vi "set point count.vi"(8 "reset":bool, 9 "dt(s)":dbl, 10 "speed":dbl) -> (1 "setpoint":dbl)   [LabVIEW 2019, in "my FPGA lib.lvlib" / "motor.lvclass"]
uses:
  motor.lvclass
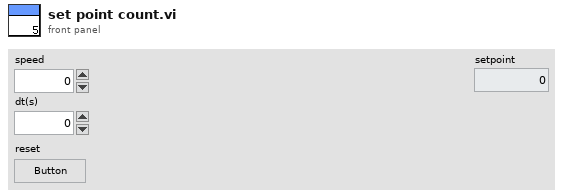
[diagram p1: front panel]
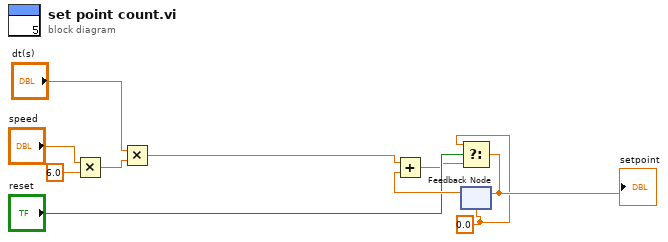
[diagram p0: block diagram]
diagram:
  w1 = 0.0
  n1 = Multiply(x="speed", y=6.0) -> (x*y=w8:dbl)
  n2 = Multiply(x="dt(s)", y=w8) -> (x*y=w4:dbl)
  n3 = feedback #1(w1) -> (w5:dbl)
  n4 = Add(x=w4, y=w5) -> (x+y=w2:dbl)
  n5 = Select(t=w1, s="reset", f=w2) -> (s? t:f=w6:dbl)
  "setpoint" <- w6
  n6 = feedback-in #1(w6) -> ()
